vi "String.Remove Quotes from String.vi"(8 "error in":errorcluster, 10 "1D String In":string[](array[string]), 11 "String In":string) -> (0 "error out":errorcluster, 2 "1D String without Quotes":string[](array[string]), 3 "String without Quotes":string)   [LabVIEW 2019]
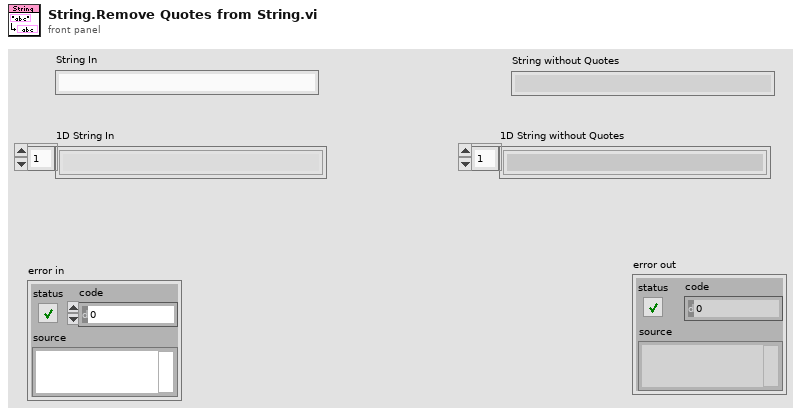
[diagram p1: front panel]
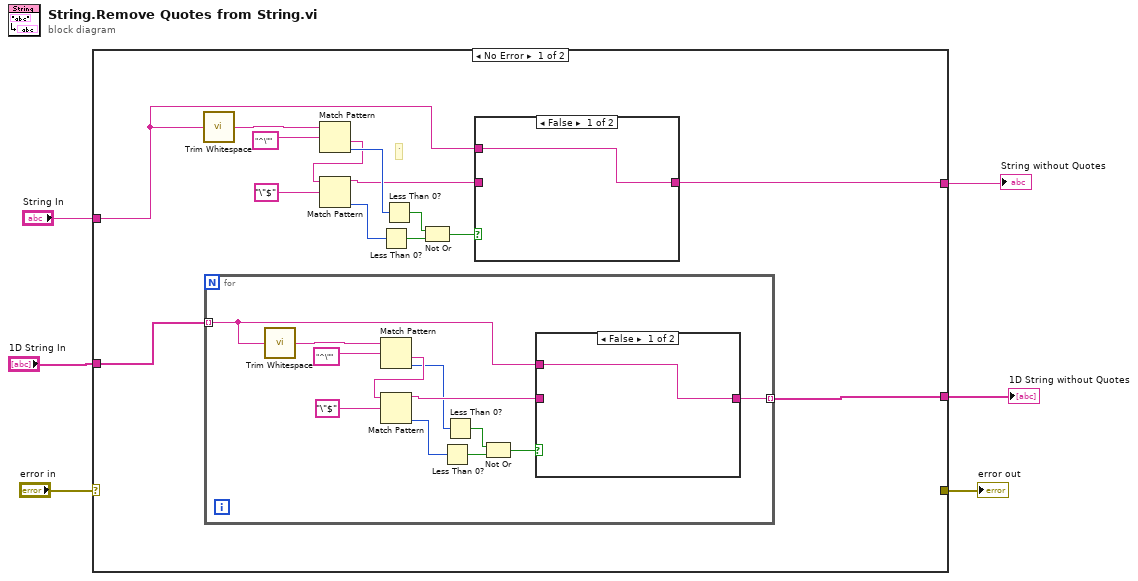
[diagram p0: block diagram]
diagram:
  n1 = case shown="No Error" "error in" {
    selector: "error in" -> [_ w37]
    tunnel: [_ w37] -> w5
    tunnel: "String In" -> [w10 _]
    tunnel: [w11 _] -> w2
    tunnel: "1D String In" -> [w8 _]
    tunnel: [w7 _] -> w1
    frame No Error {
      # "`"
      n2 = call <vilib>:"Trim Whitespace.vi"("string"=w10) -> ("trimmed string"=w9:string)  [unwired: 1 in]
      n3 = for {
        tunnel: w8 -> [w24] mode=indexing
        tunnel: [w23] -> w7 mode=indexing
        n4 = call <vilib>:"Trim Whitespace.vi"("string"=w24) -> ("trimmed string"=w34:string)  [unwired: 1 in]
        n5 = Match Pattern(string=w34, regular expression="^\"") -> (after substring=w31:string, offset past match=w27:i32)  [unwired: 1 in, 2 out]
        n6 = Match Pattern(string=w31, regular expression="\"$") -> (before substring=w33:string, offset past match=w28:i32)  [unwired: 1 in, 2 out]
        n7 = Less Than 0?(x=w28) -> (x < 0?=w29:bool)
        n8 = Less Than 0?(x=w27) -> (x < 0?=w30:bool)
        n9 = Not Or(1:w29, 2:w30) -> (0:w32:bool)
        n10 = case shown="False" w32 {
          tunnel: w33 -> [_ w36]
          tunnel: [w35 w36] -> w23
          tunnel: w24 -> [w35 _]
          frame False {
          }
          frame True {
          }
        }
      }
      n11 = Match Pattern(string=w9, regular expression="^\"") -> (after substring=w14:string, offset past match=w18:i32)  [unwired: 1 in, 2 out]
      n12 = Match Pattern(string=w14, regular expression="\"$") -> (before substring=w12:string, offset past match=w17:i32)  [unwired: 1 in, 2 out]
      n13 = Less Than 0?(x=w17) -> (x < 0?=w16:bool)
      n14 = Less Than 0?(x=w18) -> (x < 0?=w15:bool)
      n15 = Not Or(1:w16, 2:w15) -> (0:w13:bool)
      n16 = case shown="False" w13 {
        tunnel: w12 -> [_ w22]
        tunnel: [w21 w22] -> w11
        tunnel: w10 -> [w21 _]
        frame False {
        }
        frame True {
        }
      }
    }
    frame Error {
    }
  }
  "error out" <- w5
  "1D String without Quotes" <- w1
  "String without Quotes" <- w2
